vi "WSVCAP SHL FPGA LL Procedure RFFE - Receive Data.vi"(0 "Procedure Step":T1, 1 "Wait Ticks Remaining":u32, 2 "Start of Procedure":bool, 5 "RFFE Wait Ticks":u32, 7 "Read Bits Remaining":u8, 9 "Read Bytes Remaining":u8, 11 "error in (no error)":errorcluster, 12 "RFFE Cycle CMD":u64, 13 "Socket Mask":u64) -> (3 "Wait Ticks Remaining Out":u32, 4 "Procedure Step Out":T1, 6 "Read Bytes Remaining Out":u8, 8 "Read Bits Remaining Out":u8, 10 "Finished":bool, 15 "error out":errorcluster)   [LabVIEW 2012]
uses:
  Type Defs/WSVCAP SHL Procedure Step Enum.ctl
  Type Defs/WSVCAP SHL RFFE Write Line Enum.ctl
  Type Defs/WSVCAP SHL FIFO Operation Enum.ctl
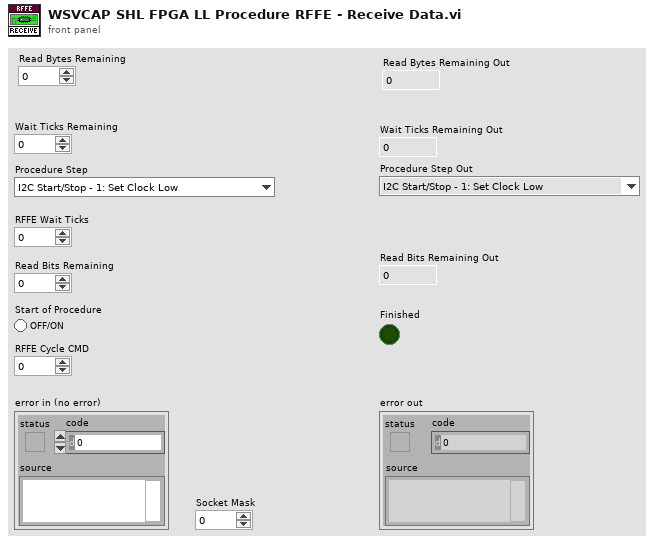
[diagram p1: front panel]
types:
  T1 = typedef "WSVCAP SHL Procedure Step Enum.ctl" = enum16{"I2C Start/Stop - 1: Set Clock Low", "I2C Start/Stop - 2: Wait", "I2C Start/Stop - 3: Set Data I", "I2C Start/Stop - 4: Wait", "I2C Start/Stop - 5: Set Clock High", "I2C Start/Stop - 6: Wait", "I2C Start/Stop - 7: Set Data II", "I2C Start/Stop - 8: Wait", "I2C Start/Stop - 9: Set Clock Low", "I2C Start/Stop - 10: Wait", "I2C Read ACK - 1: Set Clock High", "I2C Read ACK - 2: Wait", "I2C Read ACK - 3: Read ACK Bit", "I2C Read ACK - 4: Wait", "I2C Read ACK - 5: Set Clock Low", "I2C Read ACK - 6: Wait", "I2C Write ACK - 1: Write ACK Bit", "I2C Write ACK - 2: Wait", "I2C Write ACK - 3: Set Clock High", "I2C Write ACK - 4: Wait", "I2C Write ACK - 5: Set Clock Low", "I2C Write ACK - 6: Wait", "I2C Write ACK - 7: Set Data Low", "I2C Send Add - 1: Reset Bits Remaining", "I2C Send Add - 2: Set Data Bit", "I2C Send Add - 3: Wait", "I2C Send Add - 4: Set Clock High", "I2C Send Add - 5: Wait", "I2C Send Add - 6: Set Clock Low", "I2C Send Add - 7: Wait", "I2C Send Add - 8: Check Bits Remaining", "I2C Send Data - 1: Reset Bits Remaining", "I2C Send Data - 2: Load Write Bit from FIFO", "I2C Send Data - 3: Set Data Bit", "I2C Send Data - 4: Wait", "I2C Send Data - 5: Set Clock High", "I2C Send Data - 6: Wait", "I2C Send Data - 7: Set Clock Low", "I2C Send Data - 8: Wait", "I2C Send Data - 9: Check Bits Remaining", "I2C Receive Data - 1: Reset Bits Remaining", "I2C Receive Data - 2: Wait", "I2C Receive Data - 3: Set Clock High", "I2C Receive Data - 4: Wait", "I2C Receive Data - 5: Read Data Bit", "I2C Receive Data - 6: Wait", "I2C Receive Data - 7: Set Clock Low", "I2C Receive Data - 8: Wait", "I2C Receive Data - 9: Check Bits Remaining", "SPI Clear Lines - 1:Clear", "SPI Send/Receive - 1: Load SDA - Clock Low", "SPI Send/Receive - 2: Wait", "SPI Send/Receive - 3: Load DATO - Clock High", "SPI Send/Receive - 4: Wait", "SPI Wait CMD Delay - 1:Wait", "RFFE Send SSC - 1:Set Low", "RFFE Send SSC - 2:Wait", "RFFE Send SSC - 3:Set SDA High", "RFFE Send SSC - 4:Wait", "RFFE Send SSC - 5:Set SDA Low", "RFFE Send SSC - 6:Wait", "RFFE Send Data - 1:Set SCL High", "RFFE Send Data - 2:Wait", "RFFE Send Data - 3:Set SCL Low", "RFFE Send Data - 4:Wait", "RFFE Send Data - 5:Set SCL High (P)", "RFFE Send Data - 6:Wait", "RFFE Send Data - 7:Set SCL Low (P)", "RFFE Send Data - 8:Wait", "RFFE Send Data - 9:Set SCL High (BP)", "RFFE Send Data - 10:Wait", "RFFE Send Data - 11:Set SCL Low (BP)", "RFFE Send Data - 12:Wait", "RFFE Receive Data - 1:Set SCL High", "RFFE Receive Data - 2:Wait", "RFFE Receive Data - 3:Set SCL Low", "RFFE Receive Data - 4:Wait", "RFFE Receive Data - 5:Set SCL High (BP)", "RFFE Receive Data - 6:Wait", "RFFE Receive Data - 7:Set SCL Low (BP)", "RFFE Receive Data - 8:Wait", "RFFE Wait CMD Delay - 1:Wait", "RFFE Clear Lines - 1:Clear"}
  T2 = typedef "WSVCAP SHL RFFE Write Line Enum.ctl" = enum16{"SDAA", "SCLK"}
  T3 = typedef "WSVCAP SHL FIFO Operation Enum.ctl" = enum16{"Create FIFO/Memory", "Get Write FIFO Status", "Get Read FIFO Status", "Put Element in Write", "Put Element in Read", "Get Element from Write", "Get Element from Read"}
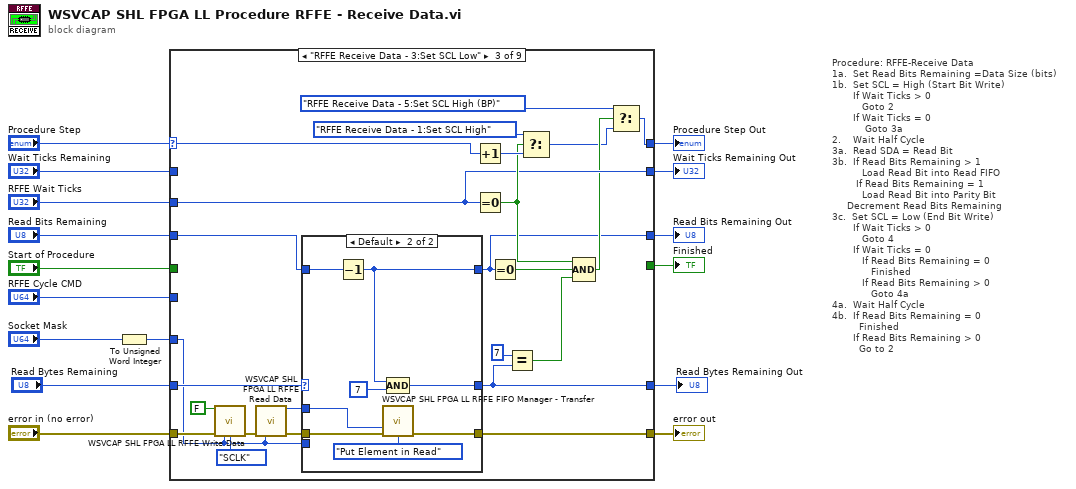
[diagram p0: block diagram]
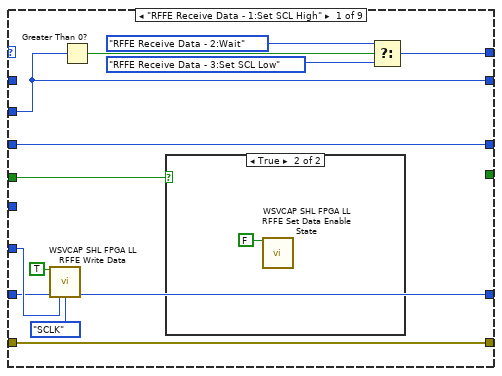
[diagram p2: hidden frame]
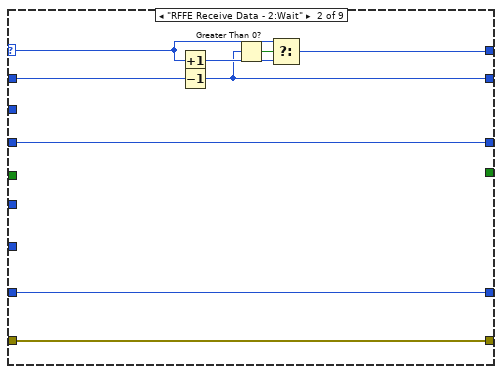
[diagram p4: hidden frame]
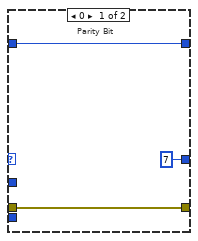
[diagram p5: hidden frame]
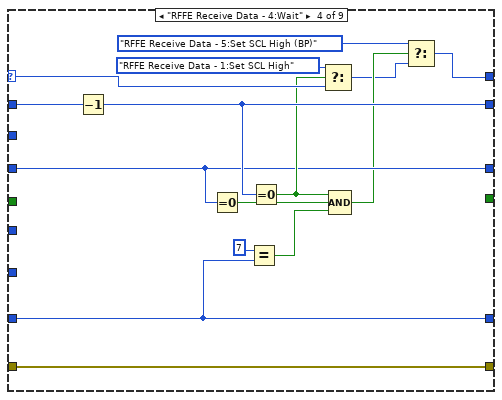
[diagram p6: hidden frame]
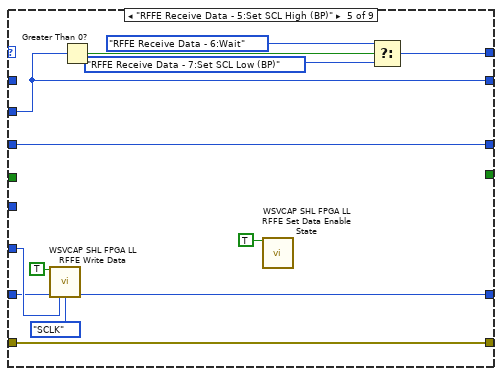
[diagram p7: hidden frame]
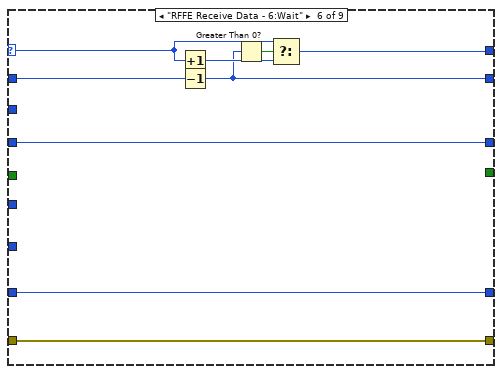
[diagram p8: hidden frame]
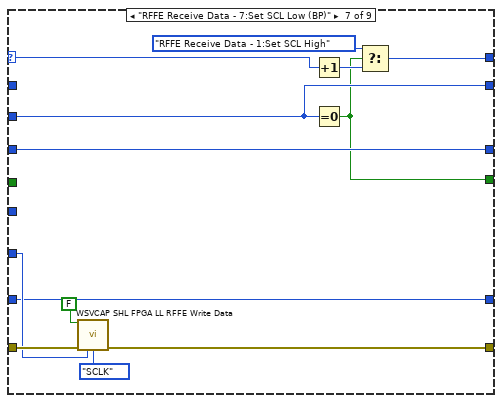
[diagram p9: hidden frame]
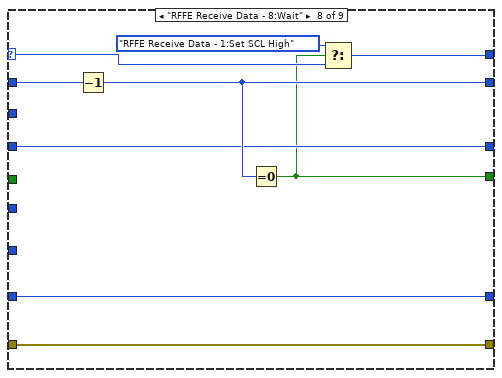
[diagram p10: hidden frame]
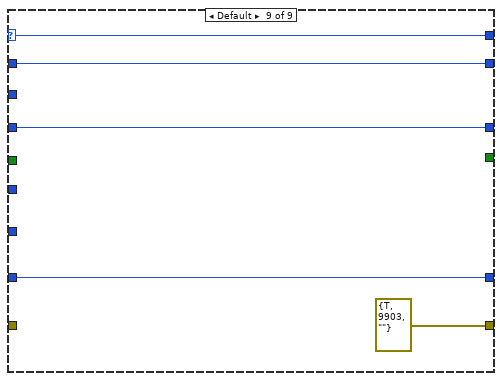
[diagram p11: hidden frame]
diagram:
  # "Procedure: RFFE-Receive Data\n1a.  Set Read Bits Remaining =Data Size (bits)\n1b.  Set SCL = High (Start Bit Write)\n       If Wait Ticks > 0\n          Goto 2\n       If Wait Ticks = 0 \n           Goto 3a\n2.    Wait Half Cycle\n3a.  Read SDA = Read Bit\n3b.  If Read Bits Remaining > 1\n          Load Read Bit into Read FIFO\n        If Read Bits Remaining = 1\n          Load Read Bit into Parity Bit\n     Decrement Read Bits Remaining\n3c.  Set SCL = Low (End Bit Write)\n       If Wait Ticks > 0\n          Goto 4\n       If Wait Ticks = 0\n          If Read Bits Remaining = 0\n             Finished\n          If Read Bits Remaining > 0\n             Goto 4a\n4a.  Wait Half Cycle\n4b.  If Read Bits Remaining = 0\n         Finished\n       If Read Bits Remaining > 0\n         Go to 2"
  n1 = To Unsigned Word Integer(number="Socket Mask") -> (unsigned 16bit integer=w12:u16)
  n2 = case shown="\"RFFE Receive Data - 3:Set SCL Low\"" "Procedure Step" {
    selector: "Procedure Step" -> [_ w36 w62 w87 _ w107 w122 w130 w135]
    tunnel: [w25 w38 w57 w88 w97 w109 w113 w131 errorcluster {"status"=TRUE, "code"=9903, "source"=""} ("error IO")] -> w15
    tunnel: "error in (no error)" -> [w25 w38 w58 w88 w97 w109 w118 w131 _]
    tunnel: "Wait Ticks Remaining" -> [_ w34 _ w86 _ w105 _ w129 w134]
    tunnel: "RFFE Wait Ticks" -> [w21 _ w53 _ w93 _ w114 _ _]
    tunnel: [_ _ _ _ _ _ w111 w124 _] -> w14
    tunnel: "Read Bits Remaining" -> [w18 w31 w48 w81 w90 w102 w112 w125 w133]
    tunnel: w12 -> [w20 _ w39 _ w92 _ w117 _ _]
    tunnel: "RFFE Cycle CMD" -> [_ _ _ _ _ _ _ _ _]
    tunnel: [w22 w33 w49 w77 w94 w104 w115 w127 w135] -> w6
    tunnel: [w21 w32 w53 w83 w93 w103 w114 w126 w134] -> w5
    tunnel: [w18 w31 w46 w81 w90 w102 w112 w125 w133] -> w4
    tunnel: "Start of Procedure" -> [w19 _ _ _ _ _ _ _ _]
    tunnel: "Read Bytes Remaining" -> [w17 w30 w47 w75 w89 w101 w110 w123 w132]
    tunnel: [w17 w30 w45 w75 w89 w101 w110 w123 w132] -> w1
    frame "RFFE Receive Data - 1:Set SCL High" {
      n3 = call "WSVCAP SHL FPGA LL RFFE Write Data.vi"("CLK In"=TRUE ("Bit In"), "Socket Mask"=w20, "Line"=WSVCAP_SHL_RFFE_Write_Line_Enum."SCLK") -> ()  [unwired: 12 in, 1 out]
      n4 = Greater Than 0?(x=w21) -> (x > 0?=w26:bool)
      n5 = case shown="True" w19 {
        frame False {
        }
        frame True {
          n6 = call "WSVCAP SHL FPGA LL RFFE Set Data Enable State.vi"("State"=FALSE) -> ()  [unwired: 14 in, 1 out]
        }
      }
      n7 = Select(t=WSVCAP_SHL_Procedure_Step_Enum."RFFE Receive Data - 2:Wait" ("Procedure Step"), s=w26, f=WSVCAP_SHL_Procedure_Step_Enum."RFFE Receive Data - 3:Set SCL Low" ("Procedure Step")) -> (s? t:f=w22:T1)
    }
    frame "RFFE Receive Data - 2:Wait" {
      n8 = Increment(x=w36) -> (x+1=w35:T1)
      n9 = Decrement(x=w34) -> (x-1=w32:u32)
      n10 = Greater Than 0?(x=w32) -> (x > 0?=w37:bool)
      n11 = Select(t=w36, s=w37, f=w35) -> (s? t:f=w33:T1)
    }
    frame "RFFE Receive Data - 3:Set SCL Low" {
      n12 = call "WSVCAP SHL FPGA LL RFFE Write Data.vi"("CLK In"=FALSE ("Bit In"), "error in (no error)"=w58, "Socket Mask"=w39, "Line"=WSVCAP_SHL_RFFE_Write_Line_Enum."SCLK") -> ("error out"=w42:errorcluster)  [unwired: 11 in]
      n13 = call "WSVCAP SHL FPGA LL RFFE Read Data.vi"("error in (no error)"=w42, "Socket Mask"=w39) -> ("Word Out (1-Bit for Each Channel)"=w40:u16, "error out"=w41:errorcluster)  [unwired: 12 in]
      n14 = case shown="Default" w47 {
        tunnel: w41 -> [w65 w67]
        tunnel: [w65 w73] -> w57
        tunnel: w39 -> [_ _]
        tunnel: w48 -> [w64 w71]
        tunnel: [w64 w69] -> w46
        tunnel: [u8 7 w68] -> w45
        tunnel: w40 -> [_ w66]
        frame 0 {
          # "Parity Bit"
        }
        frame Default {
          n15 = Decrement(x=w71) -> (x-1=w69:u8)
          n16 = call "WSVCAP SHL FPGA LL RFFE FIFO Manager - Transfer.vi"("Word In"=w66, "error in (no error)"=w67, "Operation"=WSVCAP_SHL_FIFO_Operation_Enum."Put Element in Read") -> ("error out"=w73:errorcluster)  [unwired: 10 in, 2 out]
          n17 = Compound Arithmetic op=AND(w69, u8 7 ("y")) -> (w68:u8)
        }
      }
      n18 = Increment(x=w62) -> (x+1=w61:T1)
      n19 = Equal To 0?(x=w53) -> (x = 0?=w55:bool)
      n20 = Equal To 0?(x=w46) -> (x = 0?=w56:bool)
      n21 = Equal?(x=u8 7, y=w45) -> (x = y?=w43:bool)
      n22 = Select(t=WSVCAP_SHL_Procedure_Step_Enum."RFFE Receive Data - 1:Set SCL High" ("Procedure Step"), s=w55, f=w61) -> (s? t:f=w50:T1)
      n23 = Compound Arithmetic op=AND(w55, w56, w43) -> (w52:bool)
      n24 = Select(t=WSVCAP_SHL_Procedure_Step_Enum."RFFE Receive Data - 5:Set SCL High (BP)" ("Procedure Step"), s=w52, f=w50) -> (s? t:f=w49:T1)
    }
    frame "RFFE Receive Data - 4:Wait" {
      n25 = Decrement(x=w86) -> (x-1=w83:u32)
      n26 = Equal To 0?(x=w81) -> (x = 0?=w85:bool)
      n27 = Equal?(x=u8 7, y=w75) -> (x = y?=w74:bool)
      n28 = Equal To 0?(x=w83) -> (x = 0?=w82:bool)
      n29 = Select(t=WSVCAP_SHL_Procedure_Step_Enum."RFFE Receive Data - 1:Set SCL High" ("Procedure Step"), s=w82, f=w87) -> (s? t:f=w78:T1)
      n30 = Compound Arithmetic op=AND(w82, w85, w74) -> (w80:bool)
      n31 = Select(t=WSVCAP_SHL_Procedure_Step_Enum."RFFE Receive Data - 5:Set SCL High (BP)" ("Procedure Step"), s=w80, f=w78) -> (s? t:f=w77:T1)
    }
    frame "RFFE Receive Data - 5:Set SCL High (BP)" {
      n32 = call "WSVCAP SHL FPGA LL RFFE Write Data.vi"("CLK In"=TRUE ("Bit In"), "Socket Mask"=w92, "Line"=WSVCAP_SHL_RFFE_Write_Line_Enum."SCLK") -> ()  [unwired: 12 in, 1 out]
      n33 = Greater Than 0?(x=w93) -> (x > 0?=w98:bool)
      n34 = call "WSVCAP SHL FPGA LL RFFE Set Data Enable State.vi"("State"=TRUE) -> ()  [unwired: 14 in, 1 out]
      n35 = Select(t=WSVCAP_SHL_Procedure_Step_Enum."RFFE Receive Data - 6:Wait" ("Procedure Step"), s=w98, f=WSVCAP_SHL_Procedure_Step_Enum."RFFE Receive Data - 7:Set SCL Low (BP)" ("Procedure Step")) -> (s? t:f=w94:T1)
    }
    frame "RFFE Receive Data - 6:Wait" {
      n36 = Increment(x=w107) -> (x+1=w106:T1)
      n37 = Decrement(x=w105) -> (x-1=w103:u32)
      n38 = Greater Than 0?(x=w103) -> (x > 0?=w108:bool)
      n39 = Select(t=w107, s=w108, f=w106) -> (s? t:f=w104:T1)
    }
    frame "RFFE Receive Data - 7:Set SCL Low (BP)" {
      n40 = call "WSVCAP SHL FPGA LL RFFE Write Data.vi"("CLK In"=FALSE ("Bit In"), "error in (no error)"=w118, "Socket Mask"=w117, "Line"=WSVCAP_SHL_RFFE_Write_Line_Enum."SCLK") -> ("error out"=w113:errorcluster)  [unwired: 11 in]
      n41 = Increment(x=w122) -> (x+1=w121:T1)
      n42 = Equal To 0?(x=w114) -> (x = 0?=w111:bool)
      n43 = Select(t=WSVCAP_SHL_Procedure_Step_Enum."RFFE Receive Data - 1:Set SCL High" ("Procedure Step"), s=w111, f=w121) -> (s? t:f=w115:T1)
    }
    frame "RFFE Receive Data - 8:Wait" {
      n44 = Decrement(x=w129) -> (x-1=w126:u32)
      n45 = Equal To 0?(x=w126) -> (x = 0?=w124:bool)
      n46 = Select(t=WSVCAP_SHL_Procedure_Step_Enum."RFFE Receive Data - 1:Set SCL High" ("Procedure Step"), s=w124, f=w130) -> (s? t:f=w127:T1)
    }
    frame Default {
    }
  }
  "error out" <- w15
  "Finished" <- w14
  "Procedure Step Out" <- w6
  "Wait Ticks Remaining Out" <- w5
  "Read Bits Remaining Out" <- w4
  "Read Bytes Remaining Out" <- w1
